vi "Read Encoder Position.vi"(11 "Encoder in":refnum<class "Encoder.lvclass">) -> (2 "Encoder Position":dbl[unit], 3 "Encoder out":refnum<class "Encoder.lvclass">)   [LabVIEW 2013, in "Encoder.lvclass"]
uses:
  Encoder.lvclass
  Encoder.lvclass/Encoder.ctl
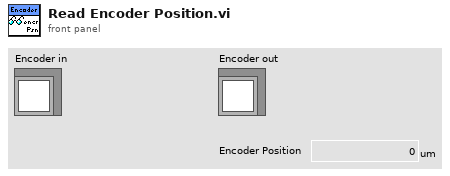
[diagram p1: front panel]
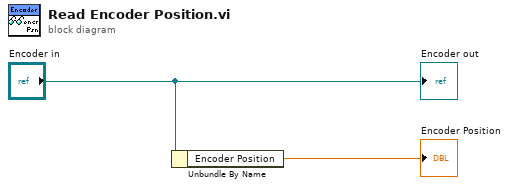
[diagram p0: block diagram]
diagram:
  n1 = Unbundle By Name("Encoder in") -> ("Encoder Position"=→"Encoder Position":dbl[unit])
  "Encoder out" <- "Encoder in"
